vi "init.vi"(8 "error in (no error)":errorcluster, 10 "VISA resource name":refnum<visa-resource-name>, 11 "3_amp_volt in":refnum<class "3_amp_volt.lvclass">) -> (0 "error out":errorcluster, 3 "3_amp_volt out":refnum<class "3_amp_volt.lvclass">)   [LabVIEW 2018, in "3_amp_volt.lvclass"]
uses:
  3_amp_volt.lvclass
  3_amp_volt.lvclass/3_amp_volt.ctl
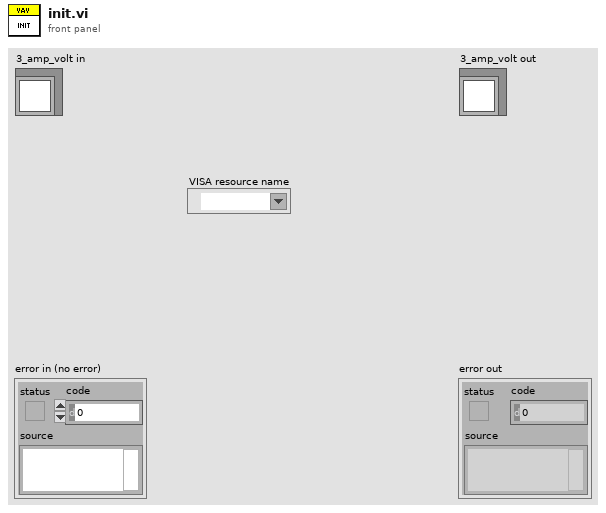
[diagram p1: front panel]
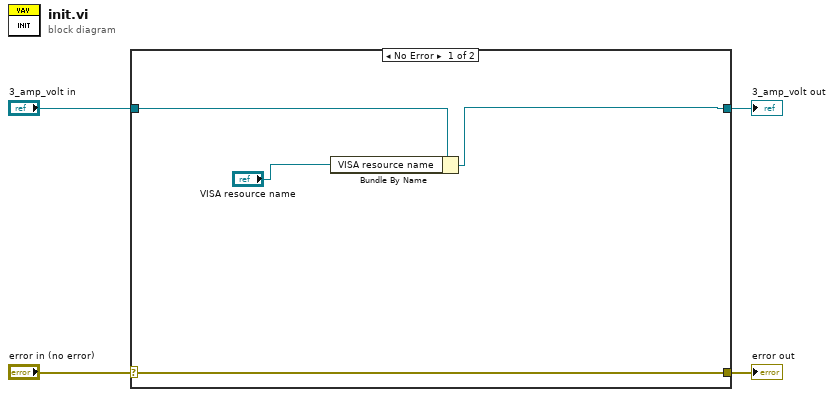
[diagram p0: block diagram]
diagram:
  n1 = case shown="No Error" "error in (no error)" {
    selector: "error in (no error)" -> [w8 w10]
    tunnel: [w8 w10] -> w3
    tunnel: [w5 w9] -> w1
    tunnel: "3_amp_volt in" -> [w7 w9]
    frame No Error {
      n2 = Bundle By Name(cluster=w7, "VISA resource name"="VISA resource name") -> (w5:refnum<class "3_amp_volt.lvclass">)
    }
    frame Error {
    }
  }
  "error out" <- w3
  "3_amp_volt out" <- w1
